vi "Error List.vi"   [LabVIEW 2015, in "QControl Creation.lvclass"]
doc: "<b> </b> <b> </b>\n©2016 Q Software Innovations, LLC (QSI)\nwritten by Quentin Alldredge\nproduced in LabVIEW 2015\n\nsupport@qsoftwareinnovations.com\nwww.qsoftwareinnovations.com\n\nAll rights reserved.\n\nRedistribution and use in source and binary forms, with or without modification, are permitted provided that the following conditions are met:\n\n * Redistributions of source code must retain the above copyright notice, this list of conditions and the following disclaimer.\n * Redistributions in binary form must reproduce the above copyright notice, this list of conditions and the following disclaimer in the documentation and/or other materials provided with the distribution.\n * Neither the name of Q Software Innovations, LLC. nor the names of its contributors may be used to endorse or promote products derived from this software without specific prior written permission.\n\nTHIS SOFTWARE IS PROVIDED BY THE COPYRIGHT HOLDERS AND CONTRIBUTORS \"AS IS\" AND ANY EXPRESS OR IMPLIED WARRANTIES, INCLUDING, BUT NOT LIMITED TO, THE IMPLIED WARRANTIES OF MERCHANTABILITY AND FITNESS FOR A PARTICULAR PURPOSE ARE DISCLAIMED. IN NO EVENT SHALL THE COPYRIGHT OWNER OR CONTRIBUTORS BE LIABLE FOR ANY DIRECT, INDIRECT, INCIDENTAL, SPECIAL, EXEMPLARY, OR CONSEQUENTIAL DAMAGES (INCLUDING, BUT NOT LIMITED TO, PROCUREMENT OF SUBSTITUTE GOODS OR SERVICES; LOSS OF USE, DATA, OR PROFITS; OR BUSINESS INTERRUPTION) HOWEVER CAUSED AND ON ANY THEORY OF LIABILITY, WHETHER IN CONTRACT, STRICT LIABILITY, OR TORT (INCLUDING NEGLIGENCE OR OTHERWISE) ARISING IN ANY WAY OUT OF THE USE OF THIS SOFTWARE, EVEN IF ADVISED OF THE POSSIBILITY OF SUCH DAMAGE."
uses:
  QControl Creation.lvclass
  <vilib>/Utility/error.llb/Error Cluster From Error Code.vi
  <vilib>/ErrorRing/Error Ring.xnode
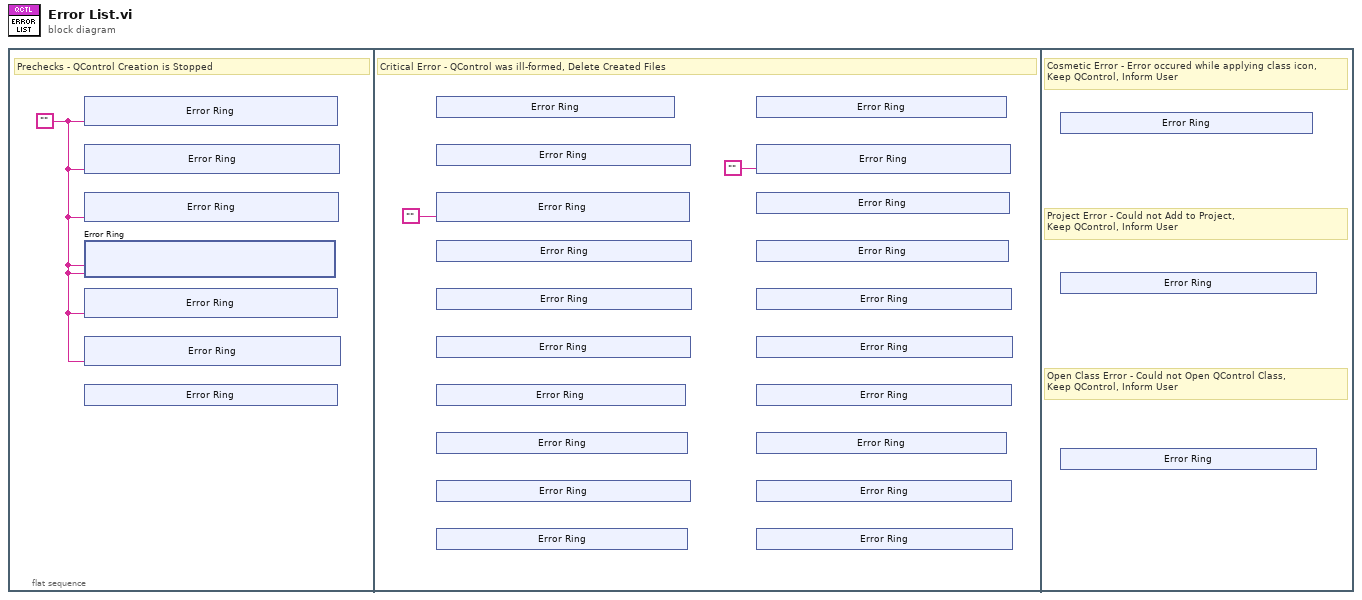
[diagram p0: block diagram]
diagram:
  n1 = flat-sequence {
    frame #0 {
      w1 = ""
      # "Prechecks - QControl Creation is Stopped"
      n2 = xnode "Error Ring"("parameter 0"=w1) -> ()  [unwired: 1 out]
      n3 = xnode "Error Ring"("parameter 0"=w1) -> ()  [unwired: 1 out]
      n4 = xnode "Error Ring"("parameter 0"=w1) -> ()  [unwired: 1 out]
      n5 = xnode "Error Ring"("parameter 0"=w1, "parameter 1"=w1) -> ()  [unwired: 1 out]
      n6 = xnode "Error Ring"("parameter 0"=w1) -> ()  [unwired: 1 out]
      n7 = xnode "Error Ring"("parameter 0"=w1) -> ()  [unwired: 1 out]
      n8 = xnode "Error Ring"() -> ()  [unwired: 1 out]
    }
    frame #1 {
      # "Critical Error - QControl was ill-formed, Delete Created Files"
      n9 = xnode "Error Ring"() -> ()  [unwired: 1 out]
      n10 = xnode "Error Ring"() -> ()  [unwired: 1 out]
      n11 = xnode "Error Ring"("parameter 0"="") -> ()  [unwired: 1 out]
      n12 = xnode "Error Ring"() -> ()  [unwired: 1 out]
      n13 = xnode "Error Ring"() -> ()  [unwired: 1 out]
      n14 = xnode "Error Ring"() -> ()  [unwired: 1 out]
      n15 = xnode "Error Ring"() -> ()  [unwired: 1 out]
      n16 = xnode "Error Ring"() -> ()  [unwired: 1 out]
      n17 = xnode "Error Ring"() -> ()  [unwired: 1 out]
      n18 = xnode "Error Ring"() -> ()  [unwired: 1 out]
      n19 = xnode "Error Ring"() -> ()  [unwired: 1 out]
      n20 = xnode "Error Ring"("parameter 0"="") -> ()  [unwired: 1 out]
      n21 = xnode "Error Ring"() -> ()  [unwired: 1 out]
      n22 = xnode "Error Ring"() -> ()  [unwired: 1 out]
      n23 = xnode "Error Ring"() -> ()  [unwired: 1 out]
      n24 = xnode "Error Ring"() -> ()  [unwired: 1 out]
      n25 = xnode "Error Ring"() -> ()  [unwired: 1 out]
      n26 = xnode "Error Ring"() -> ()  [unwired: 1 out]
      n27 = xnode "Error Ring"() -> ()  [unwired: 1 out]
      n28 = xnode "Error Ring"() -> ()  [unwired: 1 out]
    }
    frame #2 {
      # "Open Class Error - Could not Open QControl Class, \nKeep QControl, Inform User"
      # "Project Error - Could not Add to Project, \nKeep QControl, Inform User"
      # "Cosmetic Error - Error occured while applying class icon,\nKeep QControl, Inform User"
      n29 = xnode "Error Ring"() -> ()  [unwired: 1 out]
      n30 = xnode "Error Ring"() -> ()  [unwired: 1 out]
      n31 = xnode "Error Ring"() -> ()  [unwired: 1 out]
    }
  }
